vi "Boolean2String.vi"(5 "input 1":bool) -> (2 "resulting string":string)   [LabVIEW 2011]
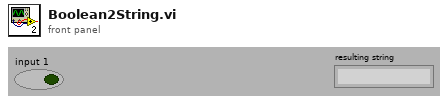
[diagram p1: front panel]
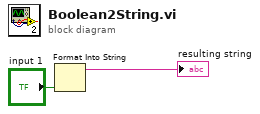
[diagram p0: block diagram]
diagram:
  n1 = Format Into String("input 1") -> (resulting string=→"resulting string":string)  [unwired: 3 in, 1 out]
